vi "Set G05 Delay.vi"(0 "Channel":u32(ring)=1 items=["T"=1, "A"=2, "B"=3], 1 "Polarity":bool=TRUE, 2 "High Drive":bool, 5 "Delay (µs)":dbl, 7 "Triggers":u32=1, 9 "Active":bool=TRUE, 11 "error in (no error)":errorcluster, 12 "Terminate":bool=TRUE, 13 "DG Number":i32) -> (15 "error out":errorcluster)   [LabVIEW 2009]
doc: "long Set_G05_Delay(unsigned long Channel, double FireFirst, unsigned long OutputModulo, BOOL Active, BOOL Positive, BOOL Terminate, BOOL HighDrive, long DG_Number);"
uses:
  BME DLL/DelayGenerator.dll
panel:
  # "NOTICE -- YOU MUST LEAVE THIS NOTICE IN PLACE.  PER THE TERMS OF THE LICENSE BELOW, YOU MAY SUBLICENSE THIS SOFTWARE \nIN ANY WAY THAT DOES NOT CONFLICT WITH THIS LICENSE.\n\n### BSD License (http://www.opensource.org/licenses/bsd-license.php) Begin ###\n \nCopyright (c) 2011, Applied Energetics, http://www.appliedenergetics.com,\n                               Richard Schwerdtfeger, <rschwerdtfeger@appliedenergetics.com>\n\nAll rights reserved.\n\nRedistribution and use in source and binary forms, with or without modification, are permitted provided that the \nfollowing conditions are met:\n\n    * Redistributions of source code must retain the above copyright notice, this list of conditions and the following disclaimer.\n    * Redistributions in binary form must reproduce the above copyright notice, this list of conditions and the following disclaimer \n       in the documentation and/or other materials provided with the distribution.\n    * Neither the name of Richard Schwerdtfeger, Applied Energetics, Inc., nor the names of its contributors may be used to \n       endorse or promote products derived from this software without specific prior written permission.\n\nTHIS SOFTWARE IS PROVIDED BY THE COPYRIGHT HOLDERS AND CONTRIBUTORS \"AS IS\" AND ANY EXPRESS OR IMPLIED WARRANTIES, \nINCLUDING, BUT NOT LIMITED TO, THE IMPLIED WARRANTIES OF MERCHANTABILITY AND FITNESS FOR A PARTICULAR PURPOSE ARE \nDISCLAIMED. IN NO EVENT SHALL THE COPYRIGHT OWNER OR CONTRIBUTORS BE LIABLE FOR ANY DIRECT, INDIRECT, INCIDENTAL,\n SPECIAL, EXEMPLARY, OR CONSEQUENTIAL DAMAGES (INCLUDING, BUT NOT LIMITED TO, PROCUREMENT OF SUBSTITUTE GOODS OR \nSERVICES; LOSS OF USE, DATA, OR PROFITS; OR BUSINESS INTERRUPTION) HOWEVER CAUSED AND ON ANY THEORY OF LIABILITY, \nWHETHER IN CONTRACT, STRICT LIABILITY, OR TORT (INCLUDING NEGLIGENCE OR OTHERWISE) ARISING IN ANY WAY OUT OF THE USE \nOF THIS SOFTWARE, EVEN IF ADVISED OF THE POSSIBILITY OF SUCH DAMAGE.\n\n### BSD License End ###"
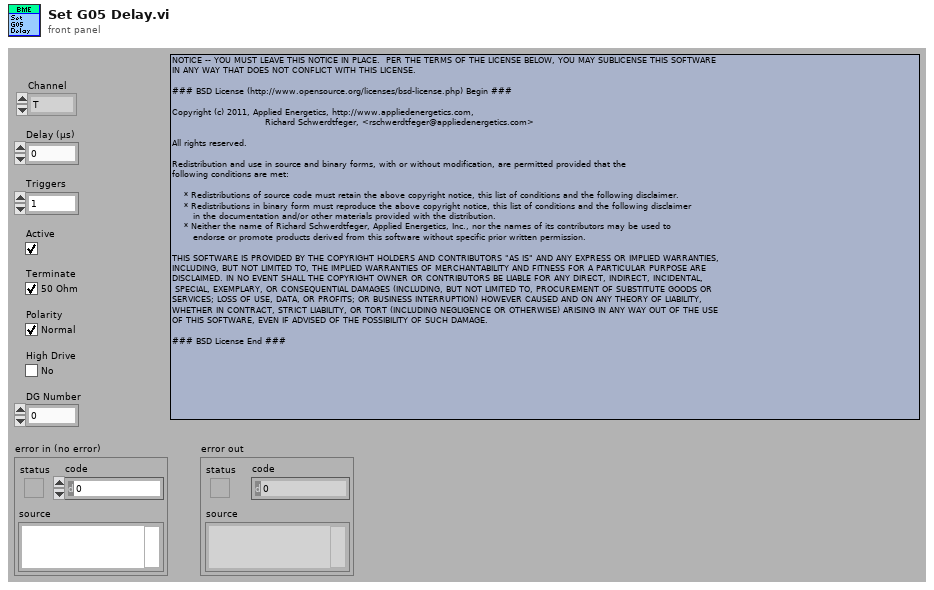
[diagram p1: front panel]
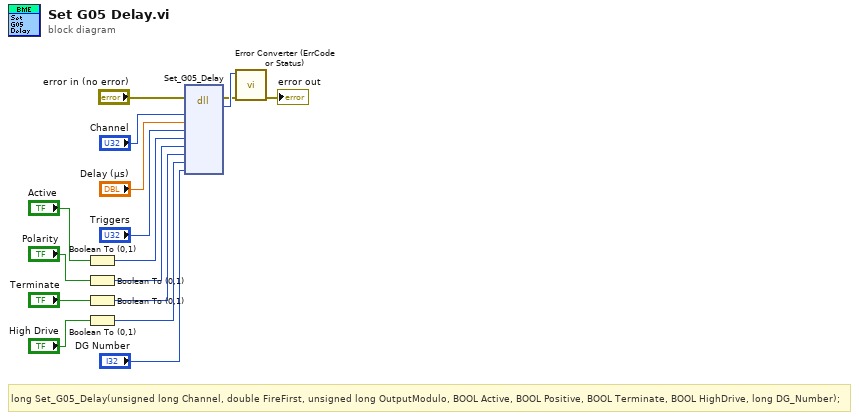
[diagram p0: block diagram]
diagram:
  # "long Set_G05_Delay(unsigned long Channel, double FireFirst, unsigned long OutputModulo, BOOL Active, BOOL Positive, BOOL Terminate, BOOL HighDrive, long DG_Number);"
  n1 = Boolean To (0,1)(Boolean="Active") -> (0, 1=w7:i16)
  n2 = Boolean To (0,1)(Boolean="Polarity") -> (0, 1=w6:i16)
  n3 = Boolean To (0,1)(Boolean="Terminate") -> (0, 1=w3:i16)
  n4 = Boolean To (0,1)(Boolean="High Drive") -> (0, 1=w1:i16)
  n5 = dll-call lib="C:/Dokumente und Einstellungen/A2.5/Desktop/POLARIS BME DG/BME DLL/DelayGenerator.*" fn="Set_G05_Delay"(error in="error in (no error)", "Channel"="Channel", "FireFirst"="Delay (µs)", "OutputModulo"="Triggers", "Active"=w7, "Positive"=w6, "Terminate"=w3, "HighDrive"=w1, "DG_Number"="DG Number") -> (error out=w10:errorcluster, w16:i32)  [unwired: 6 in, 5 out]
  n6 = call "Error Converter (ErrCode or Status).vi"("error in (no error)"=w10, "error code"=w16) -> ("error out"=→"error out":errorcluster)  [unwired: 9 out]
